vi "Test Element to Type.vi"() -> ()   [LabVIEW 2020, in "CDM-Config.lvlib"]
uses:
  CDM-Config.lvlib
  Config Manager/Config Manager.lvclass/Config Manager.ctl
  60345ea6-de85-43c0-83b6-56c5f21af443.vi
  069f57a0-40f9-48fb-a868-88c0618b894c.vi
  Config Manager/Root Element.vi
  069f57a0-40f9-48fb-a868-88c0618b894c.vi/cf897c01-1340-4b9c-857a-3ac2f60a4fa4.vi
  <vilib>/JDP Science/JSONtext/Variant to JSON Text.vi
  Config-JSON/Config From JSON.vi
  Config Element/Init.vi
  Config Element/Set Owner.vi
  Config-JSON/Element to JSON.vi
  <vilib>/JDP Science/JSONtext/JSON text to Variant.vi
  Config Element/Config Element.lvclass
  Config-JSON/Config-JSON.lvclass
  <vilib>/JDP Science/JSONtext/LVClass Serializer/JSONtext LVClass Serializer.lvclass
  Config Manager/Config Manager.lvclass
panel:
  in  "Tree":string(tree)
  out "error out":errorcluster
  out "Value":T1
  in  "Cluster":T1={"Name"="Howdy", "Numeric"=5.7, "Boolean"=TRUE, "Nested"={"Integer"=42}}
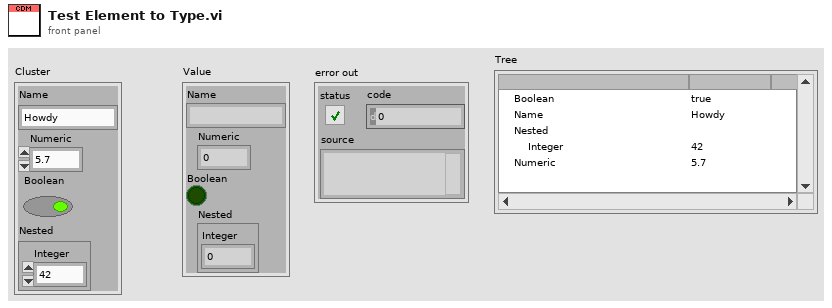
[diagram p1: front panel]
types:
  T1 = cluster{"Name":string, "Numeric":dbl, "Boolean":bool, "Nested":cluster{"Integer":i32}}
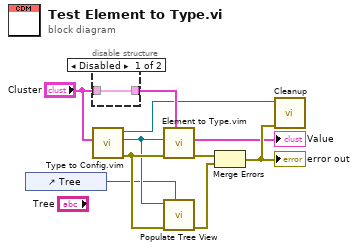
[diagram p0: block diagram]
diagram:
  n1 = control-ref of="Tree"() -> (w1:refnum<vi>)
  n2 = disable-structure shown="Disabled" {
    disable-tunnel: [w11 _] -> w7
    disable-tunnel: "Cluster" -> [w11 _]
    frame Disabled {
    }
    frame Enabled {
    }
  }
  n3 = call "Type to Config.vim"("Value"="Cluster") -> ("error out"=w9:errorcluster, "Element"=w3:refnum<class "Config Element.lvclass">, "Config"=w4:refnum<class "Config Manager.lvclass">)  [unwired: 8 in]
  n4 = call "Element to Type.vim"("Type & Defaults"=w7, "error in (no error)"=w9, "Element"=w3) -> ("error out"=w8:errorcluster, "Value"=→"Value":T1)  [unwired: 7 in]
  n5 = call "Populate Tree View.vi"("Tree"=w1, "error in (no error)"=w9, "Element"=w3) -> ("error out"=w2:errorcluster)  [unwired: 8 in]
  n6 = Merge Errors(w8, w2) -> (w10:errorcluster)
  "error out" <- w10
  n7 = call "Cleanup.vi"("error in (no error)"=w10, "Config Manager in"=w4) -> ()  [unwired: 9 in, 1 out]
